vi "Command_Velocity.vi"() -> ()   [LabVIEW 2018]
panel:
  out "Command_Velocity":dbl[](array[numeric])
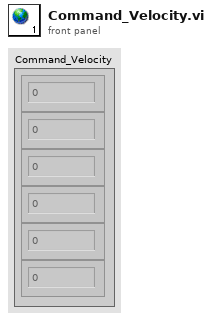
[diagram p1: front panel]
diagram:
